vi "LVIS_CalcEventResult.vi"(8 "Error In":errorcluster, 11 "TestStatus":string="*") -> (0 "Error out":errorcluster, 3 "EventInfo":T1={"EventName"="*", "EventStart"="*", "EventStop"="*", "EventStatus"="*", "EventClientID"="*", "IS_EventID"="*", "EventMeta"="*", "ProductLine"="*", "ProcessName"="*", "Station"="*", "Operator"="*", "SN"="*", "Model"="*", "Manufacturer"="*"})   [LabVIEW 2015]
doc: "Determines the event status based on all tests status."
uses:
  Globals/LVIS_IsGlobal.vi
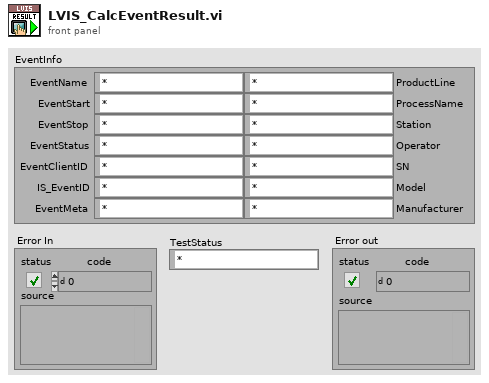
[diagram p1: front panel]
types:
  T1 = cluster{"EventName":string, "EventStart":string, "EventStop":string, "EventStatus":string, "EventClientID":string, "IS_EventID":string, "EventMeta":string, "ProductLine":string, "ProcessName":string, "Station":string, "Operator":string, "SN":string, "Model":string, "Manufacturer":string}
  T2 = cluster{"EventInfo":cluster{"EventName":string, "EventStart":string, "EventStop":string, "EventStatus":string, "EventClientID":string, "IS_EventID":string, "EventMeta":string, "ProductLine":string, "ProcessName":string, "Station":string, "Operator":string, "SN":string, "Model":string, "Manufacturer":string}, "TestInfo":cluster{"TestName":string, "TestDateTime":string, "TestStatus":string, "TestClientID":string, "IS_TestID":string, "TestMeta":string}, "MeasInfo":cluster{"MeasName":string, "MeasDateTime":string, "MeasStatus":string, "MeasClientID":string, "IS_MeasID":string, "MeasMeta":string, "MeasType":string, "MeasValue":string, "LL":string, "LL Comp":string, "HL":string, "HL Comp":string, "Units":string}}[]
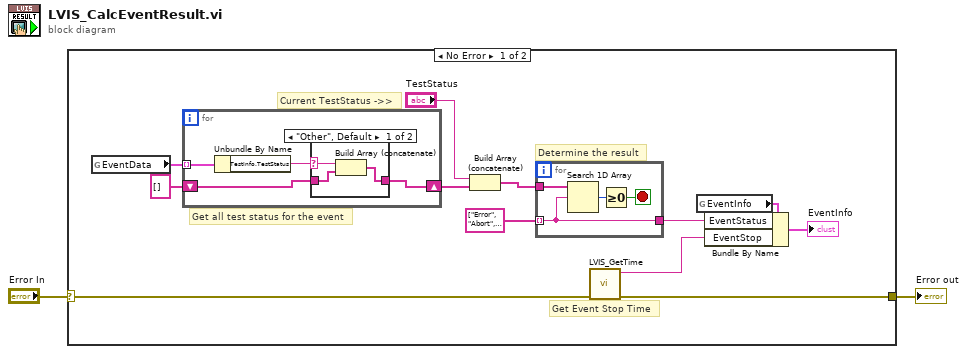
[diagram p0: block diagram]
diagram:
  n1 = case shown="No Error" "Error In" {
    selector: "Error In" -> [w5 w27]
    tunnel: [w4 w27] -> w1
    frame No Error {
      # "Get Event Stop Time"
      # "Current TestStatus ->>"
      # "Determine the result"
      # "Get all test status for the event"
      n2 = global read "LVIS_IsGlobal.vi" "EventData"() -> (w14:T2)
      n3 = for {
        tunnel: w14 -> [w22] mode=indexing
        shift-right: [w20] -> w8
        shift-left: string[] [] -> [w21]
        n4 = Unbundle By Name(w22) -> ("TestInfo.TestStatus"=w19:string)
        n5 = case shown="\"Other\", Default" w19 {
          selector: w19 -> [w23 _]
          tunnel: w21 -> [w25 w26]
          tunnel: [w24 w26] -> w20
          frame "Other", Default {
            n6 = Build Array (concatenate)(w23, w25) -> (w24:string[])
          }
          frame "Pending" {
          }
        }
      }
      n7 = Build Array (concatenate)("TestStatus", w8) -> (w7:string[])
      n8 = for {
        tunnel: w7 -> [w18]
        tunnel: string[] ["Error", "Abort", "Failed", "Passed", "Logged"] -> [w16] mode=indexing
        tunnel: [w16] -> w10
        stop <- w15 stop-if-true
        n9 = Search 1D Array(1D array=w18, element=w16) -> (index of element=w17:i32)  [unwired: 1 in]
        n10 = Greater Or Equal To 0?(x=w17) -> (x >= 0?=w15:bool)
      }
      n11 = call "LVIS_GetTime.vi"("Error In"=w5) -> ("Error out"=w4:errorcluster, "DateTime"=w3:string)  [unwired: 9 in]
      n12 = global read "LVIS_IsGlobal.vi" "EventInfo"() -> (w11:T1)
      n13 = Bundle By Name(cluster=w11, "EventStatus"=w10, "EventStop"=w3) -> (→"EventInfo":T1)
    }
    frame Error {
    }
  }
  "Error out" <- w1
